vi "Get Port Command.vi"(8 "error in (no error)":errorcluster, 9 "Puerto":string, 10 "Marca":string, 11 "Serial Device in":refnum<class "Serial Device.lvclass">) -> (0 "error out":errorcluster, 1 "Expected response":string, 2 "Command":string, 3 "Serial Device out":refnum<class "Serial Device.lvclass">)   [LabVIEW 2020, in "Serial Device.lvclass"]
uses:
  Serial Device.lvclass
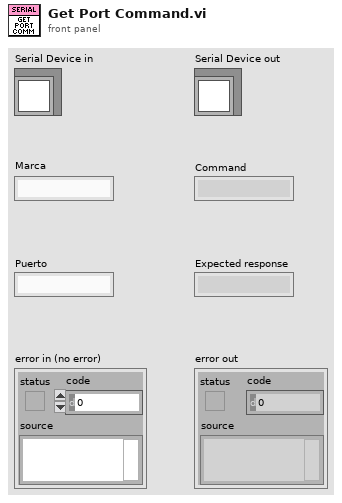
[diagram p1: front panel]
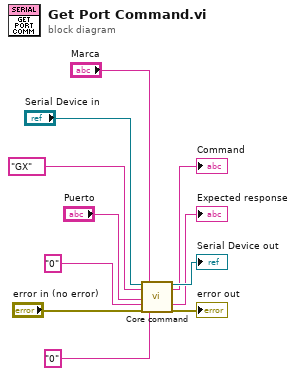
[diagram p0: block diagram]
diagram:
  n1 = call-dynamic "Core command.vi"("object in"="Serial Device in", "Command"="GX", "Param1"="Puerto", "Param2"="0", "error in (no error)"="error in (no error)", "Marca"="Marca", "Param3"="0") -> ("object out"=→"Serial Device out":refnum<class "Serial Device.lvclass">, "Command"=→"Command":string, "Expected response"=→"Expected response":string, "error out"=→"error out":errorcluster)  [unwired: 9 in]
